vi "iWorx - Event Marker.vi"() -> ()   [LabVIEW 2012]
uses:
  <vilib>/DAQmx/read.llb/DAQmx Read (Analog 1D Wfm NChan NSamp).vi
  <vilib>/DAQmx/create/channels.llb/DAQmx Create Channel (AI-Voltage-Basic).vi
  <vilib>/DAQmx/configure/timing.llb/DAQmx Timing (Sample Clock).vi
  <vilib>/DAQmx/miscellaneous.llb/DAQmx Fill In Error Info.vi
panel:
  out "Button Press Durration":dbl format="%.3f"
  in  "Set Up":bool
  out "Waveform Chart":waveform(dbl)(graph)
  in  "Snapshot":bool
  in  "Pause Button":bool
  in  "Clear Chart":bool
  out "Button Press Delta t":dbl format="%.3f"
  out "Button Press Count":u32
  in  "Reset Counter":bool
  out "Button Pressed":bool
  in  "Channel":u16(ring) items=["Channel 1", "Channel 2"]
  in  "stop":bool
  # "iWorx - Event Marker - Data Logger"
  # "Sensor Input"
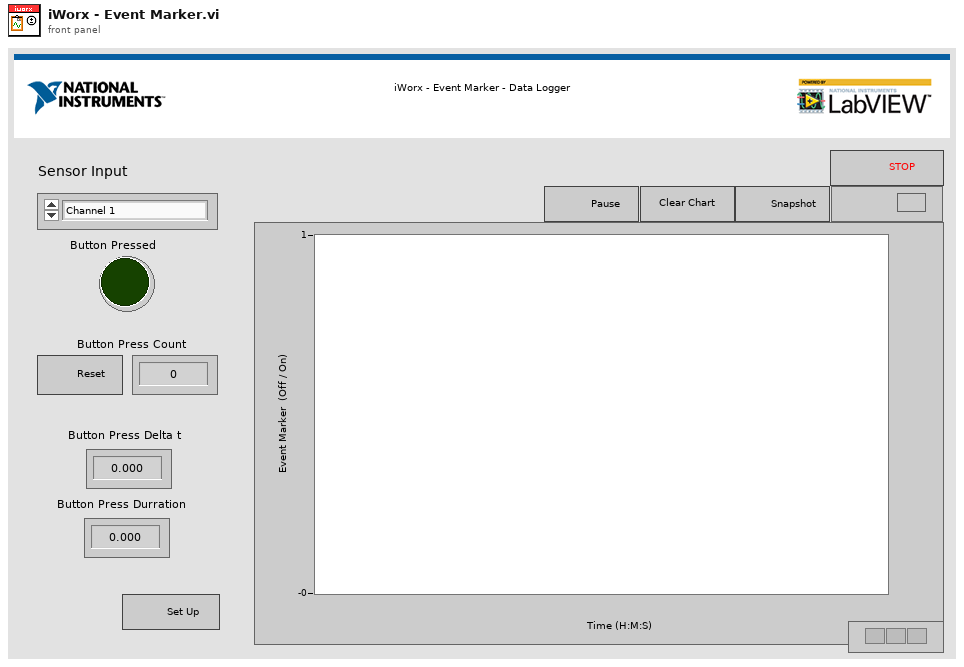
[diagram p1: front panel]
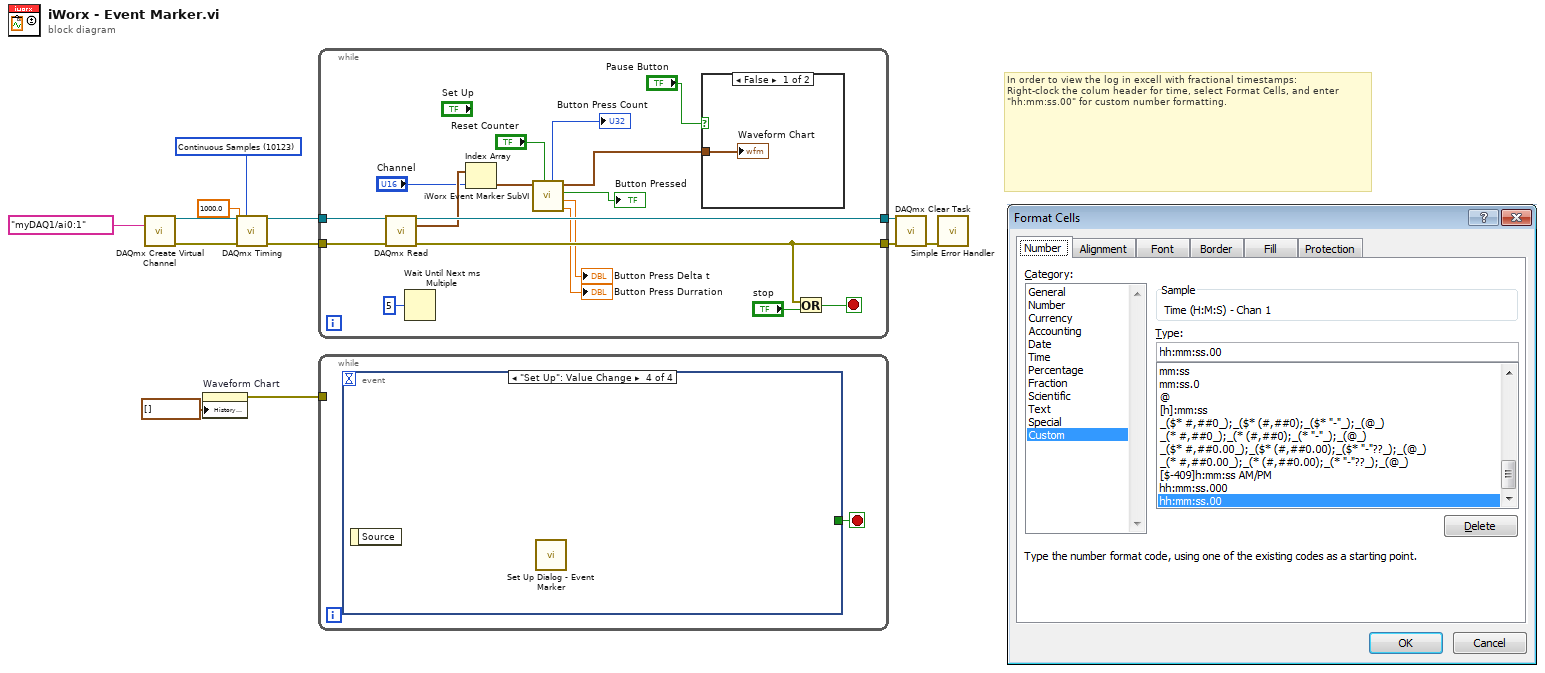
[diagram p0: block diagram]
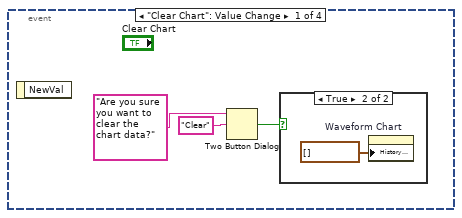
[diagram p2: hidden frame]
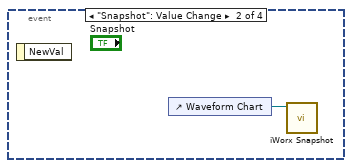
[diagram p4: hidden frame]
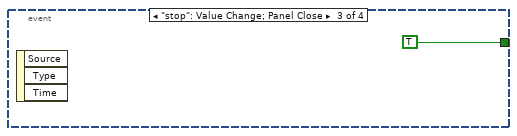
[diagram p5: hidden frame]
diagram:
  w4 = 10123 items=["Finite Samples"=10178, "Continuous Samples"=10123, "Hardware Timed Single Point"=12522] ("sample mode")
  # "In order to view the log in excell with fractional timestamps: \nRight-clock the colum header for time, select Format Cells, and enter \"hh:mm:ss.00\" for custom number formatting."
  n1 = call-poly <vilib>:"DAQmx Create Virtual Channel.vi"("physical channels"=tag "myDAQ1/ai0:1") -> ("task out"=w9:refnum<k21>, "error out"=w2:errorcluster)  [unwired: 13 in]
  n2 = property on="Waveform Chart" class="WFChart (strict)"("History Data"=waveform(dbl)[] []) -> (error out=w8:errorcluster)  [unwired: 2 in, 1 out]
  n3 = call-poly <vilib>:"DAQmx Timing.vi"("task/channels in"=w9, "sample mode"=w4, "rate"=1000.0, "error in"=w2) -> ("task out"=w5:refnum<k21>, "error out"=w1:errorcluster)  [unwired: 10 in]
  n4 = while {
    tunnel: w5 -> [w28]
    tunnel: [w27] -> w12
    tunnel: w1 -> [w26]
    tunnel: [w24] -> w11
    stop <- w25 stop-if-true
    n5 = call-poly <vilib>:"DAQmx Read.vi"("task/channels in"=w28, "error in"=w26) -> ("task out"=w27:refnum<k21>, "data"=w22:waveform(dbl)[], "error out"=w24:errorcluster)  [unwired: 11 in]
    n6 = Wait Until Next ms Multiple(millisecond multiple=u32 5) -> ()  [unwired: 1 out]
    n7 = Index Array(array=w22, index="Channel") -> (element=w18:waveform(dbl))
    n8 = call "iWorx Event Marker SubVI.vi"("Reset count (f)"="Reset Counter", "waveform in"=w18) -> ("Button Press Duration"=→"Button Press Durration":dbl, "Two Edge Separation (rising)"=→"Button Press Delta t":dbl, "Button State"=→"Button Pressed":bool, "0-1 Waveform out"=w19:waveform(dbl), "Button Count"=→"Button Press Count":u32)  [unwired: 3 in, 2 out]
    n9 = case shown="False" "Pause Button" {
      tunnel: w19 -> [w30 _]
      frame False {
        "Waveform Chart" <- w30
      }
      frame True {
      }
    }
    n10 = Or(x=w24, y="stop") -> (x .or. y?=w25:bool)
  }
  n11 = while {
    tunnel: w8 -> [_]
    stop <- w31 stop-if-true
    n12 = event shown="[3] \"Set Up\": Value Change" {
      selector: _ -> [_ _ _ _]
      dyn-events: _ -> [_ _ _ _]
      timeout: _ -> [_ _ _ _]
      tunnel: [_ _ TRUE _] -> w31
      event "Clear Chart": Value Change {
        n13 = event-data() -> ()  [unwired: 1 in, 1 out]
        n14 = Two Button Dialog(message="Are you sure you want to clear the chart data?", 2:"Clear" ("T button name (\"OK\")")) -> (T button?=w33:bool)  [unwired: 1 in]
        n15 = case shown="True" w33 {
          frame False {
          }
          frame True {
            n16 = property on="Waveform Chart" class="WFChart (strict)"("History Data"=waveform(dbl)[] []) -> ()  [unwired: 2 in, 2 out]
          }
        }
      }
      event "Snapshot": Value Change {
        n17 = event-data() -> ()  [unwired: 1 in, 1 out]
        n18 = control-ref of="Waveform Chart"() -> (w36:refnum<vi>)
        n19 = call "iWorx Snapshot.vi"("WaveformChart in"=w36) -> ()  [unwired: 10 in, 1 out]
      }
      event "stop": Value Change; Panel Close {
        n20 = event-data() -> ()  [unwired: 1 in, 3 out]
      }
      event "Set Up": Value Change {
        n21 = event-data() -> ()  [unwired: 1 in, 1 out]
        n22 = call "Set Up Dialog - Event Marker.vi"() -> ()  [unwired: 12 in]
      }
    }
  }
  n23 = call <vilib>:"DAQmx Clear Task.vi"("task in"=w12, "error in"=w11) -> ("error out"=w7:errorcluster)  [unwired: 13 in]
  n24 = call <vilib>:"Simple Error Handler.vi"("error in (no error)"=w7) -> ()  [unwired: 4 in, 5 out]
